vi "NI5112.Set special.vi"(0 "i ref in":refnum<vi>, 2 "Special":string, 3 "ms timeout (100)":i32=100, 5 "error in (no error)":errorcluster) -> (14 "i ref out":refnum<vi>, 17 "timed out":bool, 19 "error out":errorcluster)   [LabVIEW 2014, in "NI5112.lvlib"]
uses:
  NI5112.lvlib
panel:
  out "decimal integer string":string
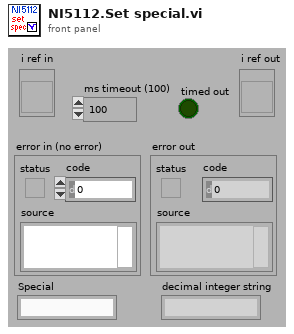
[diagram p1: front panel]
types:
  T1 = typedef "NI5112.lvlib/NI5112.i attribute.ctl" = cluster{"HWChannel":string, "instrument handle":refnum<k15>, "BinWidth":dbl, "vertical offset":dbl, "vertical range":dbl, "DataBPR":i32, "5112BPR":i32, "FullSpeed":bool, "discrLevel":dbl, "DoDiscr":bool, "VerCoupling":string}
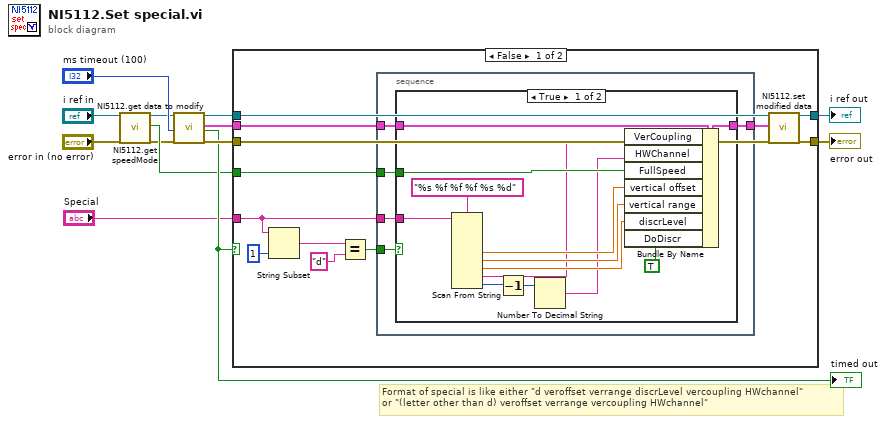
[diagram p0: block diagram]
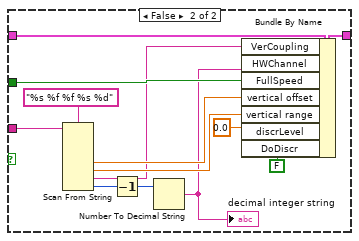
[diagram p2: hidden frame]
diagram:
  # "Format of special is like either \"d veroffset verrange discrLevel vercoupling HWchannel\"\nor \"(letter other than d) veroffset verrange vercoupling HWchannel\""
  n1 = call "NI5112.get speedMode.vi"("i ref in"="i ref in", "error in (no error)"="error in (no error)") -> ("i ref out"=w2:refnum<vi>, "fullSpeed"=w3:bool, "error out"=w1:errorcluster)  [unwired: 14 in, 1 out]
  n2 = call "NI5112.get data to modify.vi"("i ref in"=w2, "ms timeout (10000)"="ms timeout (100)", "error in (no error)"=w1) -> ("i ref out"=w11:refnum<vi>, "i attribute"=w9:T1, "timed out"=w7:bool, "error out"=w10:errorcluster)  [unwired: 13 in]
  "timed out" <- w7
  n3 = case shown="False" w7 {
    tunnel: [w25 w57] -> w13
    tunnel: [w24 w58] -> w12
    tunnel: w11 -> [w23 w58]
    tunnel: w10 -> [w22 w57]
    tunnel: w9 -> [w20 _]
    tunnel: "Special" -> [w18 _]
    tunnel: w3 -> [w19 _]
    frame False {
      n4 = String Subset(string=w18, length (rest)=1 ("length (rest)")) -> (substring=w16:string)  [unwired: 1 in]
      n5 = Equal?(x=w16, y="d") -> (x = y?=w14:bool)
      n6 = stacked-sequence {
        tunnel: [w30] -> w21
        tunnel: w20 -> [w29]
        tunnel: w19 -> [w28]
        tunnel: w18 -> [w27]
        tunnel: w14 -> [w26]
        frame #0 {
          n7 = case shown="True" w26 {
            tunnel: [w43 w56] -> w30
            tunnel: w29 -> [w42 w55]
            tunnel: w27 -> [w41 w54]
            tunnel: w28 -> [w39 w52]
            frame True {
              n8 = Scan From String(format string="%s %f %f %f %s %d", input string=w41) -> (output 2=w35:dbl, output 3=w36:dbl, output 4=w37:dbl, output 5=w34:string, output 6=w33:i32)  [unwired: 9 in, 3 out]
              n9 = Decrement(x=w33) -> (x-1=w32:i32)
              n10 = Number To Decimal String(number=w32) -> (decimal integer string=w31:string)  [unwired: 1 in]
              n11 = Bundle By Name(cluster=w42, "VerCoupling"=w34, "HWChannel"=w31, "FullSpeed"=w39, "vertical offset"=w35, "vertical range"=w36, "discrLevel"=w37, "DoDiscr"=TRUE) -> (w43:T1)
            }
            frame False {
              n12 = Scan From String(format string="%s %f %f %s %d", input string=w54) -> (output 2=w48:dbl, output 3=w49:dbl, output 4=w47:string, output 5=w46:i32)  [unwired: 8 in, 3 out]
              n13 = Decrement(x=w46) -> (x-1=w45:i32)
              n14 = Number To Decimal String(number=w45) -> (decimal integer string=w44:string)  [unwired: 1 in]
              "decimal integer string" <- w44
              n15 = Bundle By Name(cluster=w55, "VerCoupling"=w47, "HWChannel"=w44, "FullSpeed"=w52, "vertical offset"=w48, "vertical range"=w49, "discrLevel"=0.0, "DoDiscr"=FALSE) -> (w56:T1)
            }
          }
        }
      }
      n16 = call "NI5112.set modified data.vi"("i ref in"=w23, "i attribute"=w21, "error in (no error)"=w22) -> ("i ref out"=w24:refnum<vi>, "error out"=w25:errorcluster)  [unwired: 15 in]
    }
    frame True {
    }
  }
  "error out" <- w13
  "i ref out" <- w12
